vi "Update Solenoids.vi"(8 "error in (no error)":errorcluster, 11 "Robot":T1) -> (0 "error out":errorcluster)   [LabVIEW 2015]
uses:
  Robot Type Def.ctl
  <vilib>/Rock Robotics/WPI/Solenoid/WPI_SolenoidValue.ctl
  Solenoid Global.vi
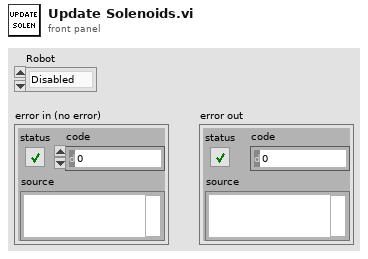
[diagram p1: front panel]
types:
  T1 = typedef "Robot Type Def.ctl" = enum32{"Disabled", "Ghost", "Casper", "Lofty", "Board", "RaceRobot", "Casper 2.0", "Excalibot 2.0"}
  T2 = typedef "WPI_SolenoidValue.ctl" = enum16{"Off", "On", "Forward", "Reverse"}
  T3 = typedef "Solenoid Type Def.ctl" = cluster{"SolenoidDevRef":cluster{"DevStatus":errorcluster, "Pneumatics Control Module":u8, "Forward Solenoid Channel":T4, "Reverse Solenoid Channel":T4}, "Open For":dbl, "Last Open":dbl}
  T4 = typedef "WPI_SolenoidChannel.ctl" = enum8{"Solenoid 0", "Solenoid 1", "Solenoid 2", "Solenoid 3", "Solenoid 4", "Solenoid 5", "Solenoid 6", "Solenoid 7", "Invalid"}
  T5 = cluster{"DevStatus":errorcluster, "Pneumatics Control Module":u8, "Forward Solenoid Channel":T4, "Reverse Solenoid Channel":T4}
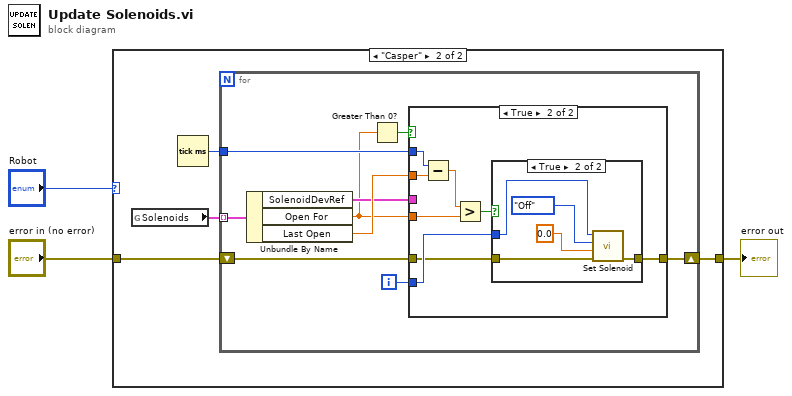
[diagram p0: block diagram]
diagram:
  n1 = case shown="\"Casper\"" "Robot" {
    tunnel: [w4 w6] -> w1
    tunnel: "error in (no error)" -> [w4 w5]
    frame Default {
    }
    frame "Casper" {
      n2 = global read "Solenoid Global.vi" "Solenoids"() -> (w8:T3[])
      n3 = Tick Count (ms)() -> (millisecond timer value=w7:u32)
      n4 = for {
        tunnel: w8 -> [w17] mode=indexing
        shift-right: [w9] -> w6
        shift-left: w5 -> [w13]
        tunnel: w7 -> [w12]
        i -> [w10]
        n5 = Unbundle By Name(w17) -> ("SolenoidDevRef"=w14:T5, "Open For"=w11:dbl, "Last Open"=w15:dbl)
        n6 = Greater Than 0?(x=w11) -> (x > 0?=w16:bool)
        n7 = case shown="True" w16 {
          tunnel: w15 -> [_ w25]
          tunnel: w14 -> [_ _]
          tunnel: w13 -> [w18 w20]
          tunnel: w12 -> [_ w26]
          tunnel: w11 -> [_ w23]
          tunnel: w10 -> [_ w21]
          tunnel: [w18 w19] -> w9
          frame False {
          }
          frame True {
            n8 = Subtract(x=w26, y=w25) -> (x-y=w24:dbl)
            n9 = Greater?(x=w24, y=w23) -> (0:w22:bool)
            n10 = case shown="True" w22 {
              tunnel: w21 -> [_ w32]
              tunnel: w20 -> [w27 w29]
              tunnel: [w27 w28] -> w19
              frame False {
              }
              frame True {
                n11 = call "Set Solenoid.vi"("error in (no error)"=w29, "On For (0 = Forever)"=0.0, "Value"=WPI_SolenoidValue."Off", "Solenoids"=w32) -> ("error out"=w28:errorcluster)  [unwired: 7 in]
              }
            }
          }
        }
      }
    }
  }
  "error out" <- w1
